vi "SetTOREG.vi"(1 "board":u32, 2 "fkt":u8) -> ()   [LabVIEW 2015]
uses:
  board.vis/ESLSCDLL.dll
panel:
  # "if (fkt==0)set to REG -> XCK\nif (fkt==1)set to REG -> OutTrig\nif (fkt==2)set to FFRead\nif (fkt==3)set to TrigIn\nif (fkt==4)set to EC\nif (fkt==5)set to DAT"
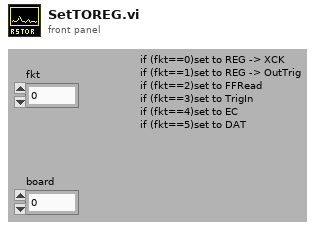
[diagram p1: front panel]
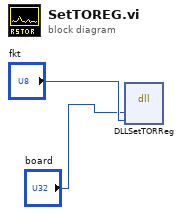
[diagram p0: block diagram]
diagram:
  n1 = dll-call lib="C:/ENTW/PCIE/64bit/lv64/lv64_eventdriven/board.vis/ESLSCDLL.dll" fn="DLLSetTORReg" ("lwlscdll.dll:DLLRsTOREG")("drv"="board", "fkt"="fkt") -> ()  [unwired: 6 in, 2 out]
